vi "Read Test Information From File.vi"(8 "error in":errorcluster, 11 "base path":path=path "C:/Gas Circulation Tester") -> (0 "error out":errorcluster, 3 "Test Configuration":T1)   [LabVIEW 2015]
uses:
  Controls/Test Configuration.ctl
  Controls/Test Information.ctl
  Controls/Vacuum Test.ctl
  Controls/Test Timing.ctl
  Controls/Vaccum Thresholds.ctl
  Controls/Helium Test.ctl
  Controls/Helium Thresholds.ctl
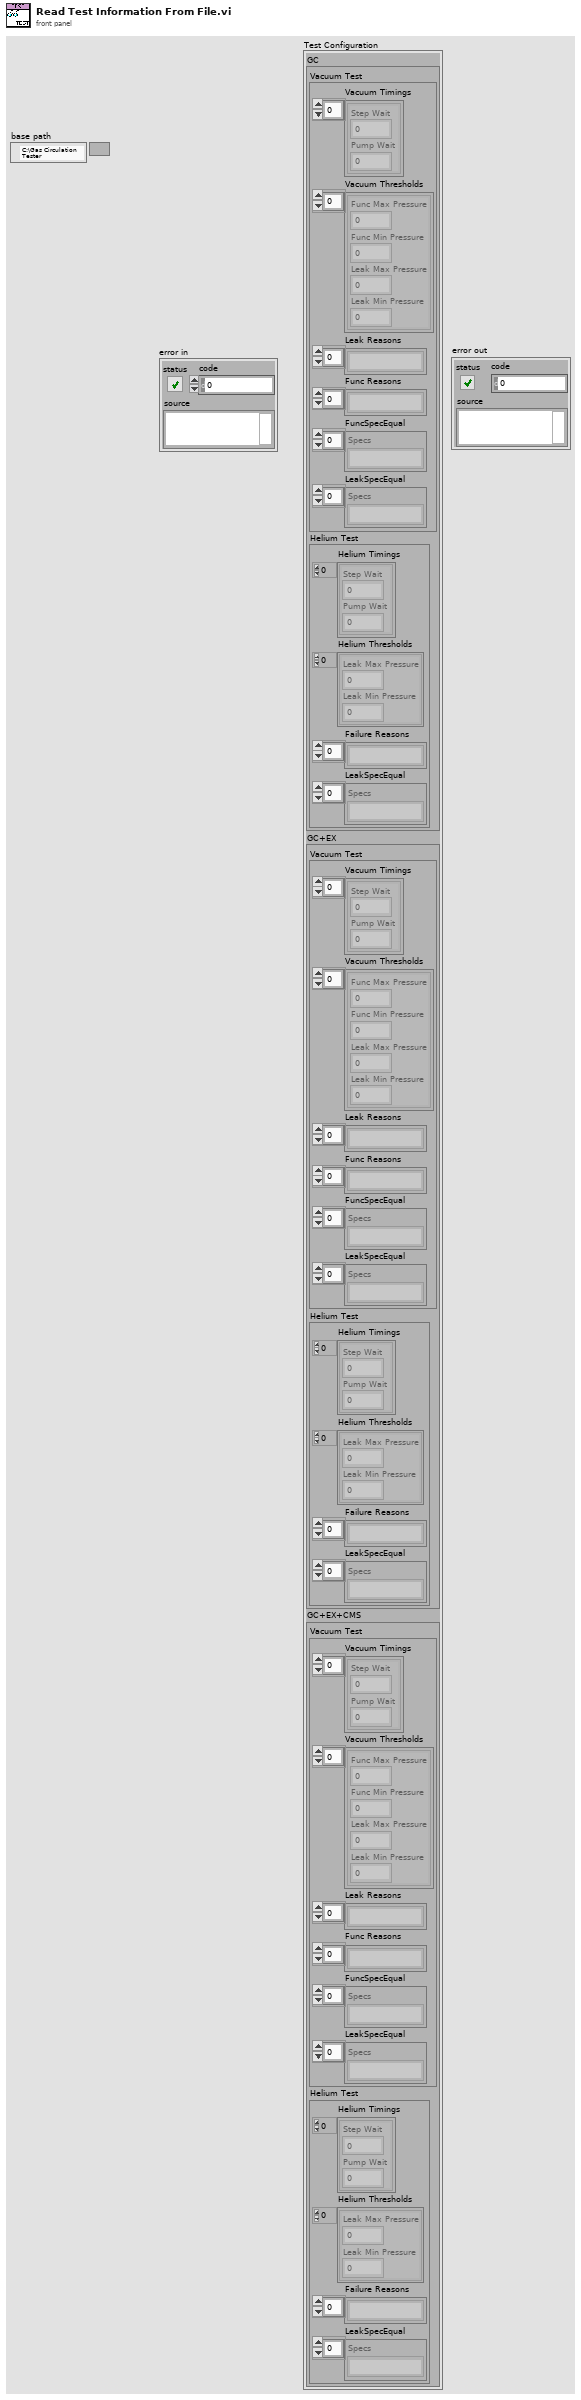
[diagram p1: front panel]
types:
  T1 = typedef "Test Configuration.ctl" = cluster{"GC":T2, "GC+EX":T2, "GC+EX+CMS":T2}
  T2 = typedef "Test Information.ctl" = cluster{"Vacuum Test":T3, "Helium Test":T6}
  T3 = typedef "Vacuum Test.ctl" = cluster{"Vacuum Timings":T4[], "Vacuum Thresholds":T5[], "Leak Reasons":string[], "Func Reasons":string[], "FuncSpecEqual":string[], "LeakSpecEqual":string[]}
  T4 = typedef "Test Timing.ctl" = cluster{"Step Wait":dbl, "Pump Wait":dbl}
  T5 = typedef "Vaccum Thresholds.ctl" = cluster{"Func Max Pressure":dbl, "Func Min Pressure":dbl, "Leak Max Pressure":dbl, "Leak Min Pressure":dbl}
  T6 = typedef "Helium Test.ctl" = cluster{"Helium Timings":T4[], "Helium Thresholds":T7[], "Failure Reasons":string[], "LeakSpecEqual":string[]}
  T7 = typedef "Helium Thresholds.ctl" = cluster{"Leak Max Pressure":dbl, "Leak Min Pressure":dbl}
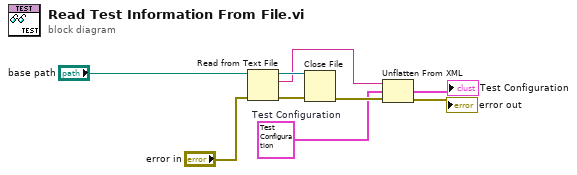
[diagram p0: block diagram]
diagram:
  w3 = T1 {"GC"={"Vacuum Test"={"Vacuum Timings"=[], "Vacuum Thresholds"=[], "Leak Reasons"=[], "Func Reasons"=[], "FuncSpecEqual"=[], "LeakSpecEqual"=[]}, "Helium Test"={"Helium Timings"=[], "Helium Thresholds"=[], "Failure Reasons"=[], "LeakSpecEqual"=[]}}, "GC+EX"={"Vacuum Test"={"Vacuum Timings"=[], "Vacuum Thresholds"=[], "Leak Reasons"=[], "Func Reasons"=[], "FuncSpecEqual"=[], "LeakSpecEqual"=[]}, "Helium Test"={"Helium Timings"=[], "Helium Thresholds"=[], "Failure Reasons"=[], "LeakSpecEqual"=[]}}, "GC+EX+CMS"={"Vacuum Test"={"Vacuum Timings"=[], "Vacuum Thresholds"=[], "Leak Reasons"=[], "Func Reasons"=[], "FuncSpecEqual"=[], "LeakSpecEqual"=[]}, "Helium Test"={"Helium Timings"=[], "Helium Thresholds"=[], "Failure Reasons"=[], "LeakSpecEqual"=[]}}}  # Test Configuration
  n1 = Read from Text File(file (use dialog)="base path", error in="error in") -> (refnum out=w8:refnum<file>, text=w7:string, error out=w9:errorcluster)  [unwired: 2 in, 1 out]
  n2 = Close File(refnum=w8, error in=w9) -> (error out=w6:errorcluster)  [unwired: 1 out]
  n3 = Unflatten From XML(xml string=w7, type=w3, error in (no error)=w6) -> (value=→"Test Configuration":T1, error out=→"error out":errorcluster)
